vi "NiFPGA Configure FIFO.vi"(8 "error in (no error)":errorcluster, 9 "Depth":u64, 10 "FIFO":u32, 11 "Session":u32) -> (0 "error out":errorcluster, 3 "Session Out":u32)   [LabVIEW 2010, in "FPGA Interface Wrapper.lvlib"]
doc: "Specifies the depth of the host memory part of the DMA FIFO. This method is optional."
uses:
  <userlib>/_FPGA Interface Advanced Tools/FPGA Interface Wrapper/FPGA Interface Wrapper.lvlib
  NiFpga.dll
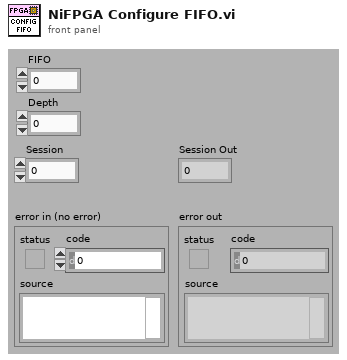
[diagram p1: front panel]
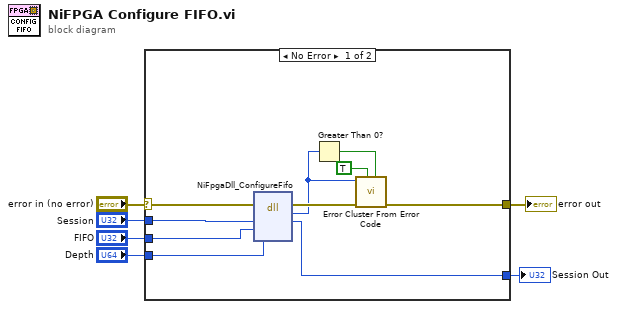
[diagram p0: block diagram]
diagram:
  n1 = case shown="No Error" "error in (no error)" {
    selector: "error in (no error)" -> [w16 w17]
    tunnel: [w7 w17] -> w5
    tunnel: "Session" -> [w15 w18]
    tunnel: [w14 w18] -> w3
    tunnel: "Depth" -> [w13 _]
    tunnel: "FIFO" -> [w12 _]
    frame No Error {
      n2 = dll-call lib="NiFpga.dll" fn="NiFpgaDll_ConfigureFifo"(error in=w16, "Session"=w15, "FIFO"=w12, "Depth"=w13) -> (error out=w9:errorcluster, "Status"=w8:i32, "Session"=w14:u32)  [unwired: 4 in, 1 out]
      n3 = Greater Than 0?(x=w8) -> (x > 0?=w10:bool)
      n4 = call <vilib>:"Error Cluster From Error Code.vi"("is warning? (False)"=w10, "show call chain? (False)"=TRUE, "error in (no error)"=w9, "error code (0)"=w8) -> ("error out"=w7:errorcluster)  [unwired: 5 in]
    }
    frame Error {
    }
  }
  "error out" <- w5
  "Session Out" <- w3
